vi "target points decide.vi"(6 "Spacing limit":i32, 8 "Y":i32, 9 "Cluster":cluster{"X":i32, "Y":i32}, 10 "X":i32) -> (2 "too close?":bool)   [LabVIEW 2014]
panel:
  out "Distance from the points set before":dbl
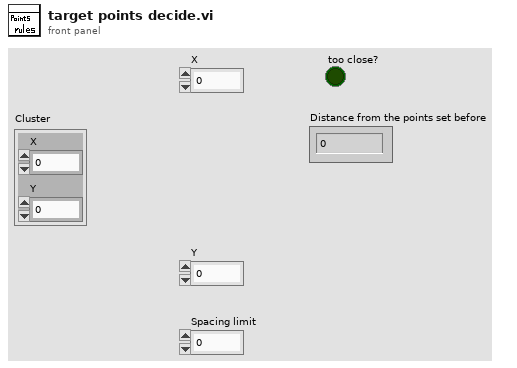
[diagram p1: front panel]
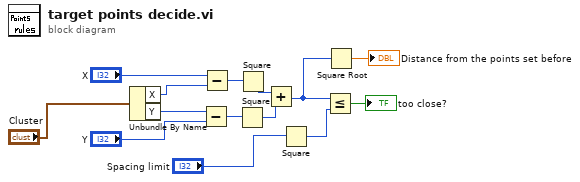
[diagram p0: block diagram]
diagram:
  n1 = Unbundle By Name("Cluster") -> ("X"=w5:i32, "Y"=w6:i32)
  n2 = Subtract(x=w6, y="Y") -> (x-y=w9:i32)
  n3 = Subtract(x="X", y=w5) -> (x-y=w8:i32)
  n4 = Square(x=w9) -> (x^2=w10:i32)
  n5 = Square(x=w8) -> (x^2=w11:i32)
  n6 = Add(x=w11, y=w10) -> (x+y=w4:i32)
  n7 = Square(x="Spacing limit") -> (x^2=w14:i32)
  n8 = Less Or Equal?(x=w4, y=w14) -> (x <= y?=→"too close?":bool)
  n9 = Square Root(x=w4) -> (sqrt(x)=→"Distance from the points set before":dbl)
